vi "Mask From Threshold.vi"(0 "image in":refnum<class "MSC Image.lvclass">, 1 "Threshold Low":dbl, 2 "Threshold High":dbl=100.0, 5 "error in (no error)":errorcluster) -> (14 "image out":refnum<class "MSC Image.lvclass">, 15 "mask image out":refnum<class "MSC Image.lvclass">, 19 "error out":errorcluster)   [LabVIEW 2016, in "MSC Image.lvclass"]
doc: "Creates a mask image from a threshold operation.\n\nLow < High: Pixels between the borders are extracted\nLow > High: Pixels excluded by the borders are extracted"
uses:
  MSC Image.lvclass
  Dependencies/x86/MSC I Process32.dll
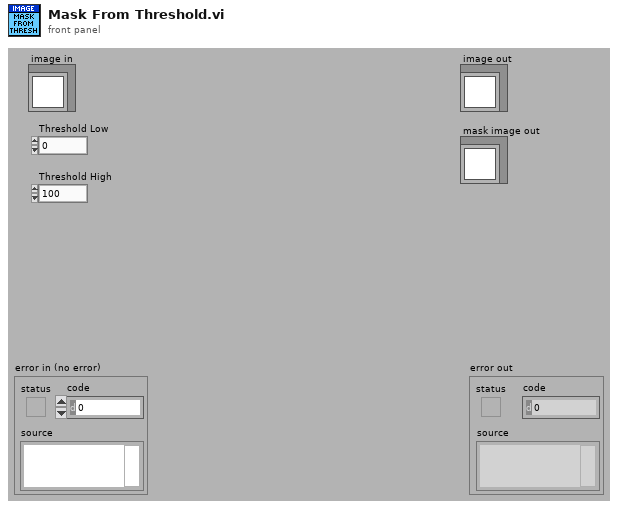
[diagram p1: front panel]
types:
  T1 = typedef "Image.ctl" = cluster{"Pointer":u64, "Size":T2, "Image Type":T3, "Time Stamp":timestamp, "Variant":variant}
  T2 = typedef "Size.ctl" = cluster{"Cols":i32, "Rows":i32}
  T3 = typedef "Image Type.ctl" = i32
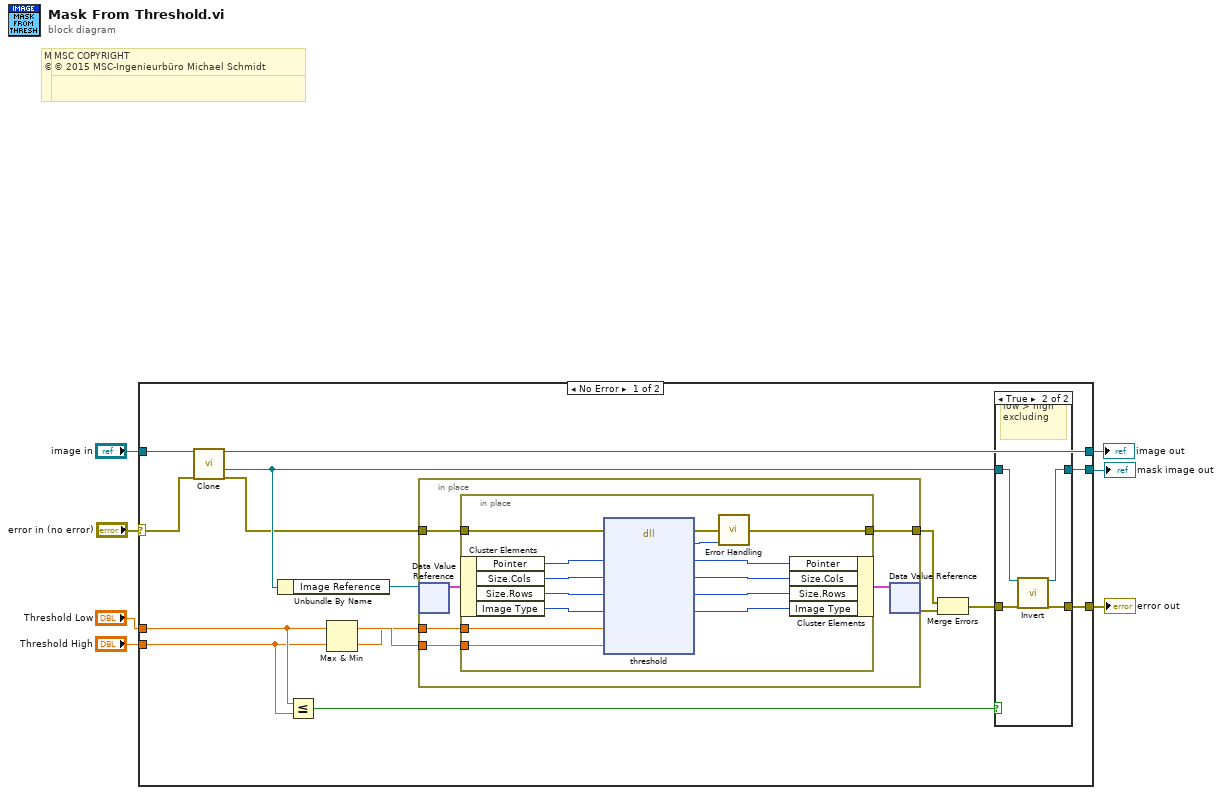
[diagram p0: block diagram]
diagram:
  # "MSC COPYRIGHT\n© 2016 MSC-Ingenieurbüro Michael Schmidt"
  # "MSC COPYRIGHT\n© 2016 MSC-Ingenieurbüro Michael Schmidt"
  # "MSC COPYRIGHT\n© 2015 MSC-Ingenieurbüro Michael Schmidt"
  # "MSC COPYRIGHT\n© 2015 MSC-Ingenieurbüro Michael Schmidt"
  n1 = case shown="No Error" "error in (no error)" {
    selector: "error in (no error)" -> [w9 w51]
    tunnel: [w13 w51] -> w6
    tunnel: "image in" -> [w12 w50]
    tunnel: [w15 _] -> w1
    tunnel: "Threshold Low" -> [w18 _]
    tunnel: "Threshold High" -> [w17 _]
    tunnel: [w11 w50] -> w2
    frame No Error {
      n2 = call-dynamic "Clone.vi"("image in"=w12, "error in (no error)"=w9) -> ("image out"=w11:refnum<class "MSC Image.lvclass">, "clone image out"=w10:refnum<class "MSC Image.lvclass">, "error out"=w8:errorcluster)  [unwired: 15 in]
      n3 = Unbundle By Name(w10) -> ("Image Reference"=w21:refnum<data-value>)
      n4 = Less Or Equal?(x=w18, y=w17) -> (x <= y?=w16:bool)
      n5 = Max & Min(x=w18, y=w17) -> (max(x,y)=w20:dbl, min(x,y)=w19:dbl)
      n6 = in-place {
        in-place-border: w8 -> [w33]
        in-place-border: [w32] -> w23
        in-place-border: w19 -> [w31]
        in-place-border: w20 -> [w30]
        n7 = in-place-dvr #1(w21) -> (w34:T1)  [unwired: 1 out]
        n8 = in-place {
          in-place-border: w33 -> [w38]
          in-place-border: [w49] -> w32
          in-place-border: w31 -> [w37]
          in-place-border: w30 -> [w36]
          n9 = in-place-cluster #2(w34) -> ("Pointer"=w48:u64, "Size.Cols"=w47:i32, "Size.Rows"=w46:i32, "Image Type"=w45:T3)
          n10 = dll-call lib="C:/Users/MSC/LabVIEW Projekte/LV 2014/MSC I-Process/user.lib/MSC-I Process/Dependencies/x86/MSC I Process*.dll" fn="threshold"(error in=w38, "pointer"=w48, "cols"=w47, "rows"=w46, "type"=w45, "thresholdLow"=w37, "thresholdHigh"=w36) -> (error out=w39:errorcluster, "error"=w40:i32, "pointer"=w44:u64, "cols"=w43:i32, "rows"=w42:i32, "type"=w41:i32)  [unwired: 4 in, 1 out]
          n11 = call "Error Handling.vi"("error in (no error)"=w39, "return type"=w40) -> ("error out"=w49:errorcluster)  [unwired: 12 in, 1 out]
          n12 = in-place-cluster #2("Pointer"=w44, "Size.Cols"=w43, "Size.Rows"=w42, "Image Type"=w41) -> (w35:T1)
        }
        n13 = in-place-dvr #1(w35) -> (w22:errorcluster)  [unwired: 1 out]
      }
      n14 = Merge Errors(w23, w22) -> (w14:errorcluster)
      n15 = case shown="True" w16 {
        tunnel: w10 -> [w25 w29]
        tunnel: [w25 w28] -> w15
        tunnel: w14 -> [w24 w27]
        tunnel: [w24 w26] -> w13
        frame False {
          # "low > high"
        }
        frame True {
          # "low > high\nexcluding"
          n16 = call-dynamic "Invert.vi"("image in"=w29, "error in (no error)"=w27) -> ("image out"=w28:refnum<class "MSC Image.lvclass">, "error out"=w26:errorcluster)  [unwired: 16 in]
        }
      }
    }
    frame Error {
    }
  }
  "error out" <- w6
  "image out" <- w2
  "mask image out" <- w1
